vi "WLAN_FrameBuild.vi"(8 "error in (no error)":errorcluster, 10 "Modulation parameter":T1, 11 "data in":i8[](array[numeric]) caption="input bit stream") -> (0 "error out":errorcluster, 3 "output array":cdb[](array[numeric]))   [LabVIEW 2014]
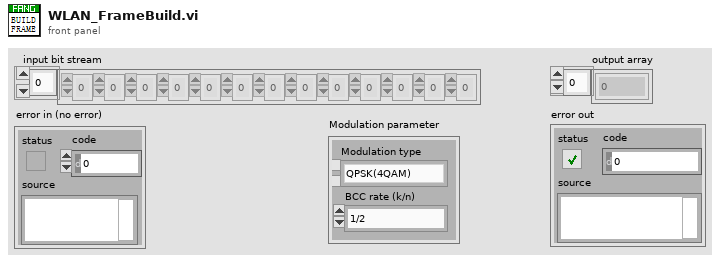
[diagram p1: front panel]
types:
  T1 = cluster{"Modulation type":enum16{"QPSK(4QAM)", "64QAM", "16QAM", "BPSK"}, "BCC rate (k/n)":enum16{"1/2", "2/3", "3/4"}}
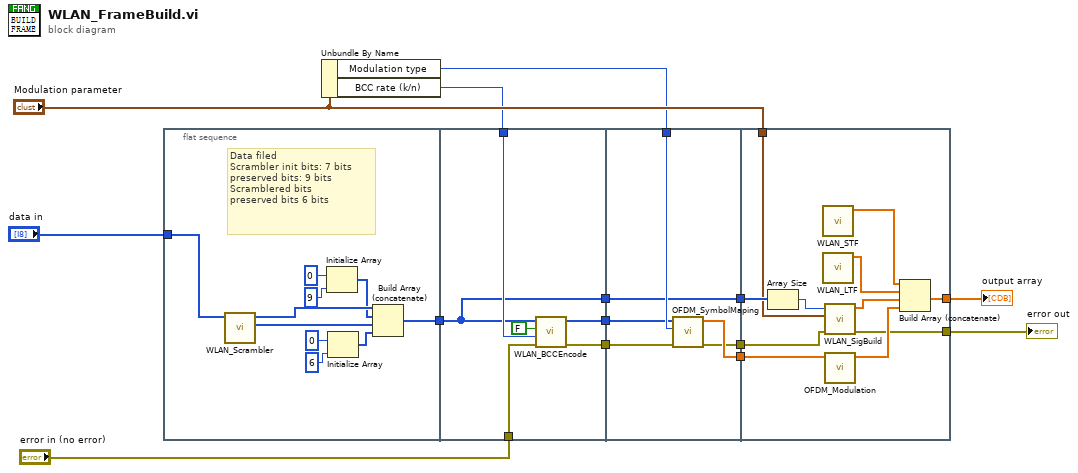
[diagram p0: block diagram]
diagram:
  n1 = flat-sequence {
    tunnel: "data in" -> [w16]
    tunnel: [w15] -> w13
    tunnel: w13 -> [w25]
    tunnel: "error in (no error)" -> [w29]
    tunnel: [w28] -> w11
    tunnel: [w27] -> w10
    tunnel: w7 -> [w26]
    tunnel: [w25] -> w2
    tunnel: w11 -> [w35]
    tunnel: w10 -> [w34]
    tunnel: w8 -> [w36]
    tunnel: [w33] -> w6
    tunnel: [w32] -> w5
    tunnel: w2 -> [w31]
    tunnel: [w31] -> w1
    tunnel: "Modulation parameter" -> [w45]
    tunnel: w6 -> [w44]
    tunnel: w5 -> [w39]
    tunnel: [w38] -> w4
    tunnel: [w37] -> w3
    tunnel: w1 -> [w47]
    frame #0 {
      # "Data filed\nScrambler init bits: 7 bits\npreserved bits: 9 bits\nScramblered bits\npreserved bits 6 bits"
      n2 = call "WLAN_Scrambler.vi"("input bit stream"=w16) -> ("scrambled bits"=w20:i8[], "scrambler initial bit"=w24:i8[])  [unwired: 9 in]
      n3 = Initialize Array(i8 0 ("element"), 9 ("dimension size")) -> (w23:i8[])
      n4 = Initialize Array(i8 0 ("element"), 6 ("dimension size")) -> (w17:i8[])
      n5 = Build Array (concatenate)(w24, w23, w20, w17) -> (w15:i8[])
    }
    frame #1 {
      n6 = call "WLAN_BCCEncode.vi"("error in (no error)"=w29, "BCC rate (k/n)"=w26, "need add zeros?"=FALSE, "input bit stream"=w25) -> ("error out"=w28:errorcluster, "output bit stream 3"=w27:i8[])  [unwired: 6 in]
    }
    frame #2 {
      n7 = call "OFDM_SymbolMaping.vi"("error in (no error)"=w35, "Modulation type"=w36, "input bit stream"=w34) -> ("error out"=w32:errorcluster, "symbols"=w33:cdb[])  [unwired: 7 in]
    }
    frame #3 {
      n8 = Array Size(array=w47) -> (size(s)=w46:i32)
      n9 = call "WLAN_STF.vi"() -> ("STF"=w40:cdb[])  [unwired: 11 in]
      n10 = call "WLAN_LTF.vi"() -> ("LTF"=w41:cdb[])  [unwired: 11 in]
      n11 = call "WLAN_SigBuild.vi"("Data bit length"=w46, "Modulation parameter"=w45, "error in (no error)"=w39) -> ("symbols"=w42:cdb[], "error out"=w38:errorcluster)  [unwired: 6 in]
      n12 = call "OFDM_Modulation.vi"("Input sequence"=w44) -> ("Output sequence"=w43:cdb[])  [unwired: 10 in]
      n13 = Build Array (concatenate)(w40, w41, w42, w43) -> (w37:cdb[])
    }
  }
  n14 = Unbundle By Name("Modulation parameter") -> ("Modulation type"=w8:enum16{"QPSK(4QAM)", "64QAM", "16QAM", "BPSK"}, "BCC rate (k/n)"=w7:enum16{"1/2", "2/3", "3/4"})
  "output array" <- w3
  "error out" <- w4
